vi "Set Controls(Buttons).vi"(3 "Button Primary":T2) -> (0 "Button Primary":bool)   [LabVIEW 2014]
uses:
  Button Actions.ctl
  SRE Enum.ctl
  Support Code/Robot Global Data.vi
panel:
  out "Button Secondary":bool
  in  "Button Secondary":T1(ring)
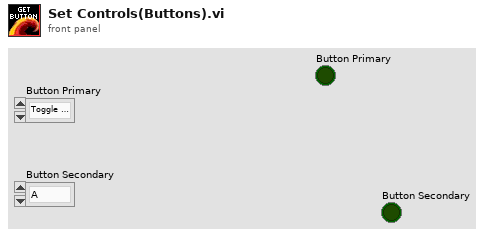
[diagram p1: front panel]
types:
  T1 = enum16{"A", "B", "X", "Y", "Left bumper", "Right bumper", "Back", "Start", "Left Joystick down", "Right Joystick down"}
  T2 = typedef "Button Actions.ctl" = enum16{"Toggle Field Centric", "Gyro Reset"}
  T3 = typedef "SRE Enum.ctl" = enum16{"Start", "Run", "End"}
  T4 = enum16{"A", "B", "X", "Y", "Left bumper", "Right bumper", "Back", "Start", "Left Joystick down", "Right Joystick down"}[]
  T5 = enum16{"Trigger Left", "2 Left", "3 Left", "4 Left", "5 Left", "6 Left", "7 Left", "8 Left", "9 Left", "10 Left", "11 Left", "Trigger Right", "2 Right", "3 Right", "4 Right", "5 Right", "6 Right", "7 Right", "8 Right", "9 Right", "10 Right", "11 Right"}[]
  T6 = enum16{"Trigger Left", "2 Left", "3 Left", "4 Left", "5 Left", "6 Left", "7 Left", "8 Left", "9 Left", "10 Left", "11 Left", "Trigger Right", "2 Right", "3 Right", "4 Right", "5 Right", "6 Right", "7 Right", "8 Right", "9 Right", "10 Right", "11 Right"}
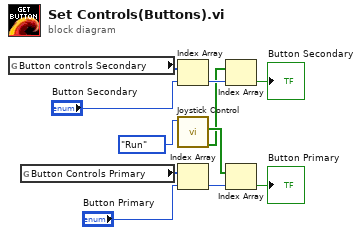
[diagram p0: block diagram]
diagram:
  n1 = global read "Robot Global Data.vi" "Button controls Secondary"() -> (w1:T4)
  n2 = global read "Robot Global Data.vi" "Button Controls Primary"() -> (w9:T5)
  n3 = Index Array(array=w1, index="Button Secondary") -> (element=w5:T1)
  n4 = call "Joystick Control.vi"("Enum"=SRE_Enum."Run") -> ("Buttons Output Secondary"=w3:bool[], "Button Output Primary"=w6:bool[])  [unwired: 5 in, 2 out]
  n5 = Index Array(array=w9, index="Button Primary") -> (element=w8:T6)
  n6 = Index Array(array=w3, index=w5) -> (element=→"Button Secondary":bool)
  n7 = Index Array(array=w6, index=w8) -> (element=→"Button Primary":bool)
